vi "Helmholtz2D_FEM_Assemble_Coef Mtrx.vi"(4 "a":dbl, 6 "k":dbl, 7 "# of unknown":i32, 8 "Mass Mtrx":dbl[][](array[numeric]), 9 "Stiffness Mtrx":dbl[][](array[numeric]), 10 "Triangle":i32[](array[numeric]), 11 "Coef Mtrx In":T1) -> (3 "Coef Mtrx Out":T1)   [LabVIEW 2020, in "NI_PDE.lvlib"]
uses:
  <vilib>/gmath/NI_PDE.lvlib
  <vilib>/gmath/pde.llb/Common/PDE_Sparse Mtrx.ctl
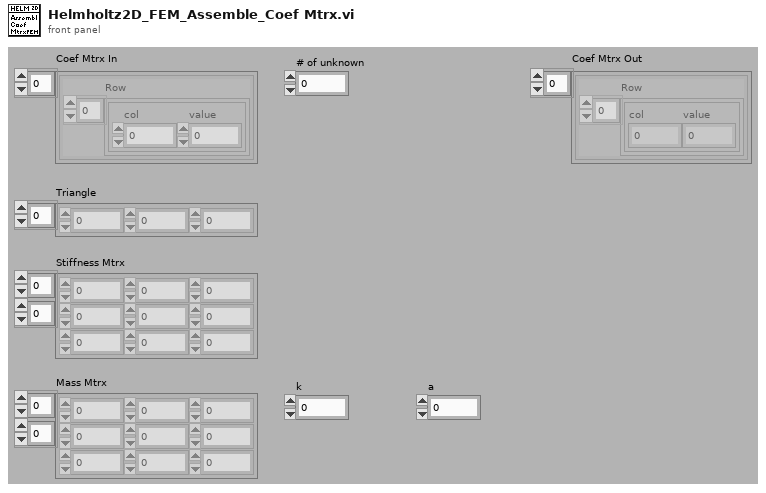
[diagram p1: front panel]
types:
  T1 = typedef "NI_PDE.lvlib/PDE_Sparse Mtrx.ctl" = cluster{"Row":cluster{"col":i32, "value":dbl}[]}[]
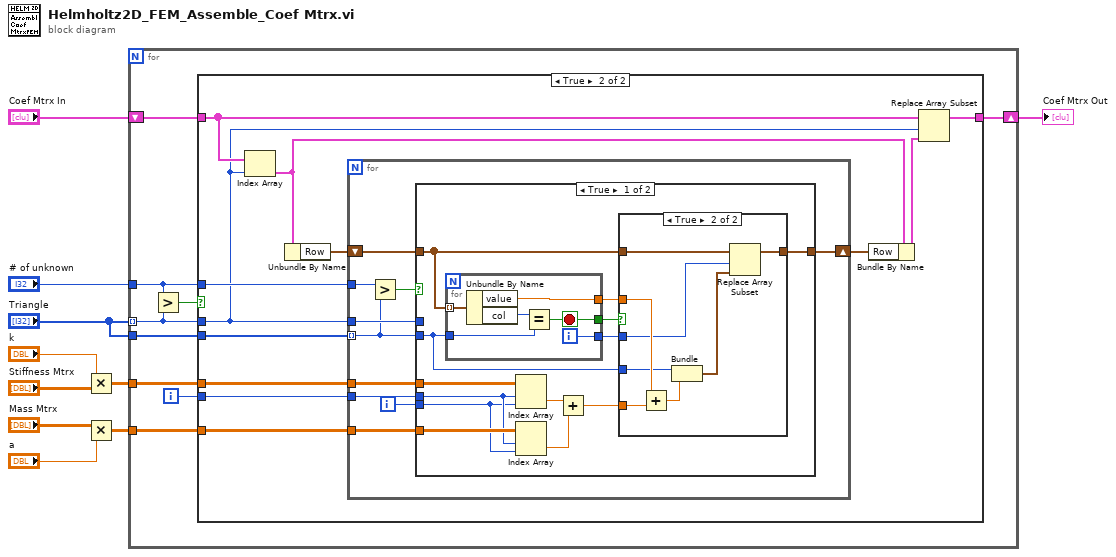
[diagram p0: block diagram]
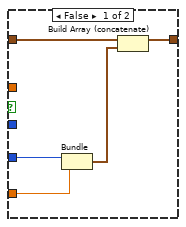
[diagram p3: hidden frame]
diagram:
  n1 = Multiply(x="k", y="Stiffness Mtrx") -> (x*y=w10:dbl[][])
  n2 = Multiply(x="Mass Mtrx", y="a") -> (x*y=w9:dbl[][])
  n3 = for {
    tunnel: "Triangle" -> [w13] mode=indexing
    tunnel: "Triangle" -> [w19]
    tunnel: w10 -> [w18]
    tunnel: w9 -> [w17]
    shift-right: [w15] -> w8
    shift-left: "Coef Mtrx In" -> [w16]
    tunnel: "# of unknown" -> [w12]
    i -> [w14]
    n4 = Greater?(x=w12, y=w13) -> (0:w11:bool)
    n5 = case shown="True" w11 {
      tunnel: w19 -> [_ w32]
      tunnel: w18 -> [_ w31]
      tunnel: w17 -> [_ w30]
      tunnel: w16 -> [w20 w26]
      tunnel: [w20 w25] -> w15
      tunnel: w14 -> [_ w29]
      tunnel: w13 -> [_ w24]
      tunnel: w12 -> [_ w28]
      frame False {
      }
      frame True {
        n6 = Index Array(array=w26, index=w24) -> (element=w23:cluster{"Row":cluster{"col":i32, "value":dbl}[]})
        n7 = Unbundle By Name(w23) -> ("Row"=w27:cluster{"col":i32, "value":dbl}[])
        n8 = for {
          tunnel: w32 -> [w35] mode=indexing
          tunnel: w24 -> [w40]
          tunnel: w31 -> [w39]
          tunnel: w30 -> [w38]
          tunnel: w28 -> [w42]
          tunnel: w29 -> [w37]
          shift-right: [w33] -> w22
          shift-left: w27 -> [w34]
          i -> [w36]
          n9 = Greater?(x=w42, y=w35) -> (0:w41:bool)
          n10 = case shown="True" w41 {
            tunnel: w40 -> [_ _]
            tunnel: w35 -> [w44 _]
            tunnel: w39 -> [w55 _]
            tunnel: w38 -> [w53 _]
            tunnel: w37 -> [w52 _]
            tunnel: w36 -> [w51 _]
            tunnel: w34 -> [w47 w75]
            tunnel: [w43 w75] -> w33
            frame True {
              n11 = for {
                tunnel: w47 -> [w74] mode=indexing
                tunnel: w44 -> [w72]
                tunnel: [w71] -> w49
                tunnel: [w70] -> w48
                tunnel: [w69] -> w46
                i -> [w70]
                stop <- w71 stop-if-true
                n12 = Unbundle By Name(w74) -> ("value"=w69:dbl, "col"=w73:i32)
                n13 = Equal?(x=w73, y=w72) -> (x = y?=w71:bool)
              }
              n14 = Index Array(array=w55, index (row)=w52, index (col)=w51) -> (element=w54:dbl)
              n15 = Index Array(array=w53, index (row)=w52, index (col)=w51) -> (element=w50:dbl)
              n16 = Add(x=w54, y=w50) -> (x+y=w45:dbl)
              n17 = case shown="True" w49 {
                tunnel: w48 -> [_ w61]
                tunnel: w47 -> [w58 w64]
                tunnel: w46 -> [_ w68]
                tunnel: w45 -> [w59 w67]
                tunnel: w44 -> [w60 w65]
                tunnel: [w56 w63] -> w43
                frame False {
                  n18 = Bundle("Numeric"=w60, w59) -> (w57:cluster{"Numeric":i32, dbl})  [unwired: 1 out]
                  n19 = Build Array (concatenate)(w58, w57) -> (w56:cluster{"Numeric":i32, "value":dbl}[])
                }
                frame True {
                  n20 = Add(x=w68, y=w67) -> (x+y=w66:dbl)
                  n21 = Bundle("Numeric"=w65, w66) -> (w62:cluster{"Numeric":i32, dbl})  [unwired: 1 out]
                  n22 = Replace Array Subset(array=w64, new element=w62, index=w61) -> (w63:cluster{"col":i32, "value":dbl}[])
                }
              }
            }
            frame False {
            }
          }
        }
        n23 = Bundle By Name(cluster=w23, "Row"=w22) -> (w21:cluster{"Row":cluster{"col":i32, "value":dbl}[]})
        n24 = Replace Array Subset(array=w26, new element=w21, index=w24) -> (w25:T1)
      }
    }
  }
  "Coef Mtrx Out" <- w8
